vi "2 angle_iteration.vi"(1 "Phi":dbl, 3 "Wind Vector":cluster{"Wind R":dbl, "Wind Theta":dbl}) -> (0 "Best Theta":dbl)   [LabVIEW 2011]
doc: "Given one angle, this VI returns a partner angle which minimizes travel time to the waypoint. It does this by checking 180 different angles and returning the optimal one."
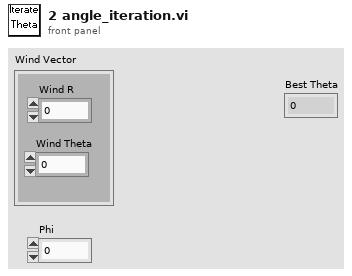
[diagram p1: front panel]
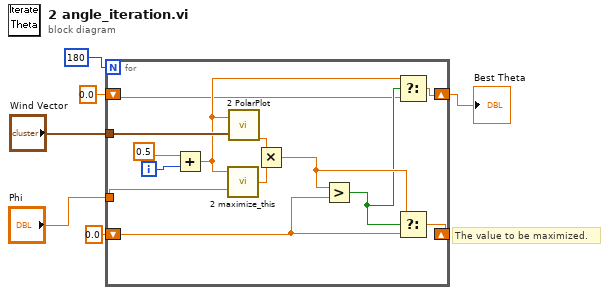
[diagram p0: block diagram]
diagram:
  # "The value to be maximized."
  n1 = for {
    N: 180 -> [_]
    tunnel: "Wind Vector" -> [w17]
    tunnel: "Phi" -> [w16]
    shift-right: [w12] -> _
    shift-left: 0.0 -> [w11]
    shift-right: [w8] -> w1
    shift-left: 0.0 -> [w7]
    i -> [w19]
    n2 = Add(x=0.5, y=w19) -> (x+y=w9:dbl)
    n3 = call "2 maximize_this.vi"("Phi"=w16, "Theta"=w9) -> ("Value"=w14:dbl)  [unwired: 1 in]
    n4 = call "2 PolarPlot.vi"("Wind Vector"=w17, "Boat Angle"=w9) -> ("Velocity"=w15:dbl)
    n5 = Multiply(x=w15, y=w14) -> (x*y=w13:dbl)
    n6 = Greater?(x=w13, y=w11) -> (0:w10:bool)
    n7 = Select(t=w9, s=w10, f=w7) -> (s? t:f=w8:dbl)
    n8 = Select(t=w13, s=w10, f=w11) -> (s? t:f=w12:dbl)
  }
  "Best Theta" <- w1
